vi "Query Options.vi"(8 "error in (no error)":errorcluster, 11 "Manual PSU in":refnum<class "Manual PSU.lvclass">) -> (0 "error out":errorcluster, 2 "Options":string[](array[string]), 3 "Manual PSU out":refnum<class "Manual PSU.lvclass">)   [LabVIEW 2020, in "Manual PSU.lvclass"]
uses:
  Manual PSU.lvclass
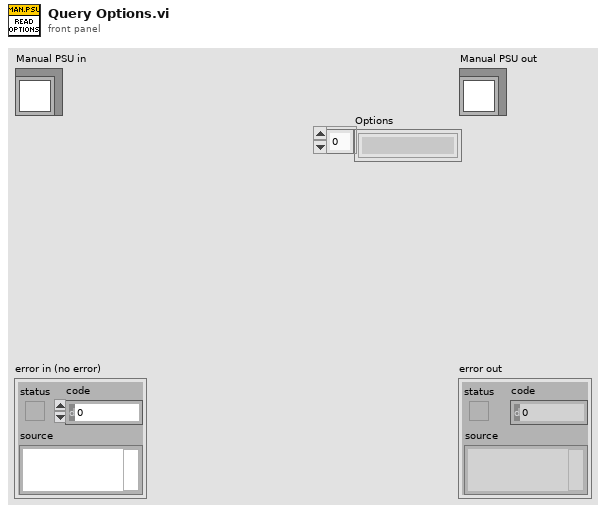
[diagram p1: front panel]
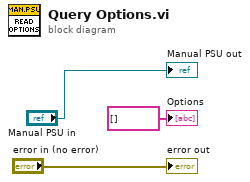
[diagram p0: block diagram]
diagram:
  "error out" <- "error in (no error)"
  "Manual PSU out" <- "Manual PSU in"
  "Options" <- string[] [] ("Options")
